vi "Readback Data_w_Waveform_no logging.vi"(0 "Semiconductor Module Context":T1, 5 "Pins":string[](array[string])=["CLK", "SDA"], 9 "Digital Format":string="RFFE6", 11 "error in (no error)":errorcluster, 12 "Register_Address_Dec":u8=80 format="%.0x", 13 "Bit_Location(LSB)":u8=7 max=7, 14 "#ofBits":u8=1 min=1 max=8) -> (4 "Reg Value":u8 format="%.0b", 15 "error out":errorcluster)   [LabVIEW 2013]
uses:
  <vilib>/NI_TestStand_SemiconductorModule/NI_TestStand_Semiconductor_Module.lvlibp/PinMap/General/SemiconductorModuleContext.ctl
  MIPI_RFFE/Ctrls/Configuration.ctl
  MIPI_RFFE/Ctrls/ClockDataChannels.ctl
  MIPI_RFFE/Ctrls/RegReadWrite.ctl
  <instrlib>/niHSDIO/niHSDIO.llb/niHSDIO_ctl Generation Mode Values (Ring).ctl
  <vilib>/NI_TestStand_SemiconductorModule/NI_TestStand_Semiconductor_Module.lvlibp/PinMap/HSDIO/PinsToNIHSDIOSessions.vi
  <vilib>/Waveform/DWDTOps.llb/DWDT Digital Size.vi
  <instrlib>/niHSDIO/niHSDIO.llb/niHSDIO Write Named Waveform (WDT).vi
  <instrlib>/niHSDIO/niHSDIO.llb/niHSDIO Fetch Waveform (WDT).vi
  <vilib>/NI_TestStand_SemiconductorModule/NI_TestStand_Semiconductor_Module.lvlibp
panel:
  out "Converted Data":T2 {"Register" max=31 format="%.0x"; "Slave Address" max=15 format="%.0x"}
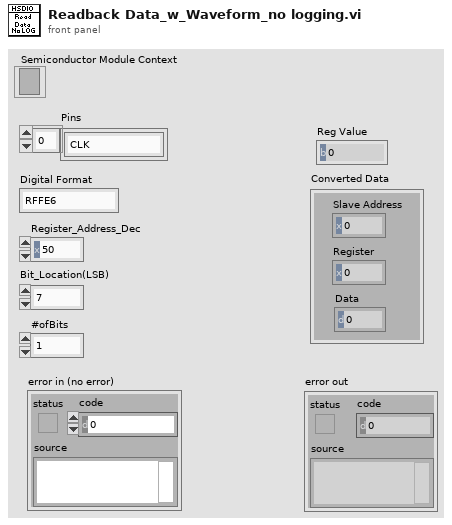
[diagram p1: front panel]
types:
  T1 = typedef "NI_TestStand_Semiconductor_Module.lvlibp/SemiconductorModuleContext.ctl" = refnum<k7>
  T2 = cluster{"Slave Address":u8, "Register":u8, "Data":u8}
  T3 = typedef "RegReadWrite.ctl" = cluster{"Slave Address":u8, "Register":u8, "Data":u8, "SetID_Pin_State":enum16{"0", "1", "Z"}}
  T4 = typedef "Configuration.ctl" = cluster{"Samples to Allocate":i32, "Oversample Factor":u8, "Clock Channel":T5, "Data Channel":T5}
  T5 = typedef "ClockDataChannels.ctl" = enum16{"0", "1"}
  T6 = typedef "niHSDIO_ctl Generation Mode Values (Ring).ctl" = i32
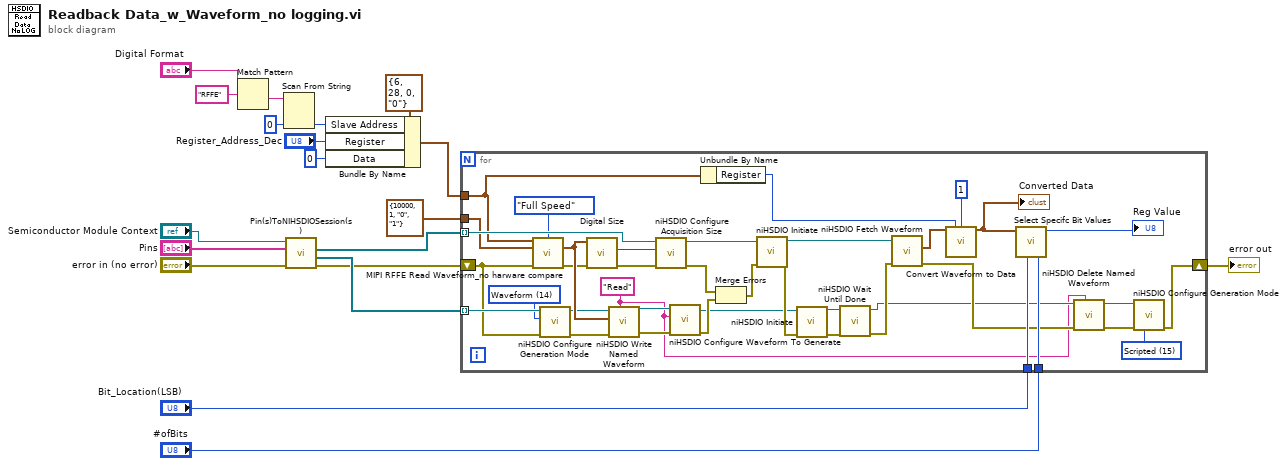
[diagram p0: block diagram]
diagram:
  n1 = Match Pattern(string="Digital Format", regular expression="RFFE") -> (after substring=w4:string)  [unwired: 1 in, 3 out]
  n2 = Scan From String(input string=w4, default 1=u8 0 ("Slave Address")) -> (output 1=w2:u8)  [unwired: 3 in, 3 out]
  n3 = call-poly <vilib>:"Pin(s)ToNIHSDIOSession(s).vi"("error in (no error)"="error in (no error)", "Pins"="Pins", "Semiconductor Module Context"="Semiconductor Module Context") -> ("error out"=w16:errorcluster, "Generation Sessions"=w17:refnum<k15>[], "Acquisition Sessions"=w18:refnum<k15>[])  [unwired: 3 in, 3 out]
  n4 = Bundle By Name(cluster=T3 {"Slave Address"=6, "Register"=28, "Data"=0, "SetID_Pin_State"=enum."0"} ("Data"), "Slave Address"=w2, "Register"="Register_Address_Dec", "Data"=u8 0) -> (w7:T3)
  n5 = for {
    tunnel: w18 -> [w48] mode=indexing
    tunnel: w17 -> [w38] mode=indexing
    tunnel: w7 -> [w27]
    tunnel: T4 {"Samples to Allocate"=10000, "Oversample Factor"=1, "Clock Channel"=enum."0", "Data Channel"=enum."1"} ("Configuratation") -> [w46]
    tunnel: "Bit_Location(LSB)" -> [w45]
    tunnel: "#ofBits" -> [w44]
    shift-right: [w29] -> w1
    shift-left: w16 -> [w35]
    w28 = T6 15 items=["Waveform"=14, "Scripted"=15] ("generation mode (waveform)")
    w20 = "Read" ("waveform name (default:\"\")")
    w34 = T6 14 items=["Waveform"=14, "Scripted"=15] ("generation mode (waveform)")
    n6 = call "MIPI RFFE Read Waveform_no harware compare.vi"("Data"=w27, "Readback Speed"=enum16{"Full Speed", "Half Speed"}."Full Speed", "Configuratation"=w46, "error in (no error)"=w35) -> ("Waveform Graph"=w53:digitalwaveform, "error out"=w50:errorcluster)  [unwired: 10 in]
    n7 = call <instrlib>:"niHSDIO Configure Generation Mode.vi"("error in (no error)"=w35, "generation mode (waveform)"=w34, "instrument handle"=w38) -> ("error out"=w36:errorcluster, "instrument handle out"=w37:refnum<k15>)  [unwired: 7 in]
    n8 = call-poly <vilib>:"Digital Size.vi"("error in (no error)"=w50, "digital waveform in"=w53) -> ("error out"=w51:errorcluster, "number of samples"=w52:i32)  [unwired: 6 in, 2 out]
    n9 = call-poly <instrlib>:"niHSDIO Write Named Waveform.vi"("waveform name (default:\"\")"=w20, "error in (no error)"=w36, "data"=w53, "instrument handle"=w37) -> ("error out"=w33:errorcluster, "instrument handle out"=w31:refnum<k15>)  [unwired: 6 in]
    n10 = call <instrlib>:"niHSDIO Configure Acquisition Size.vi"("error in (no error)"=w51, "samples per record (1000 samples)"=w52, "instrument handle"=w48) -> ("error out"=w47:errorcluster, "instrument handle out"=w55:refnum<k15>)  [unwired: 7 in]
    n11 = call <instrlib>:"niHSDIO Configure Waveform To Generate.vi"("error in (no error)"=w33, "waveform name"=w20, "instrument handle"=w31) -> ("error out"=w32:errorcluster, "instrument handle out"=w30:refnum<k15>)  [unwired: 7 in]
    n12 = Unbundle By Name(w27) -> ("Register"=w26:u8)
    n13 = Merge Errors(w47, w32) -> (w56:errorcluster)
    n14 = call <instrlib>:"niHSDIO Initiate.vi"("error in (no error)"=w56, "instrument handle"=w55) -> ("error out"=w58:errorcluster, "instrument handle out"=w39:refnum<k15>)  [unwired: 8 in]
    n15 = call <instrlib>:"niHSDIO Initiate.vi"("error in (no error)"=w58, "instrument handle"=w30) -> ("error out"=w57:errorcluster, "instrument handle out"=w40:refnum<k15>)  [unwired: 8 in]
    n16 = call <instrlib>:"niHSDIO Wait Until Done.vi"("error in (no error)"=w57, "instrument handle"=w40) -> ("error out"=w43:errorcluster, "instrument handle out"=w22:refnum<k15>)  [unwired: 8 in]
    n17 = call-poly <instrlib>:"niHSDIO Fetch Waveform.vi"("error in (no error)"=w43, "instrument handle"=w39) -> ("error out"=w24:errorcluster, "data"=w54:digitalwaveform)  [unwired: 6 in, 2 out]
    n18 = call "Convert Waveform to Data.vi"("Waveform Graph"=w54, "Register"=w26, "Ext_Read_Num_Reg"=u8 1) -> ("Converted Data"=w49:T2)  [unwired: 10 in, 2 out]
    "Converted Data" <- w49
    n19 = call "Select Specifc Bit Values.vi"("#ofBits"=w44, "Bit_Location(LSB)"=w45, "Converted Data"=w49) -> ("Bits"=→"Reg Value":u8)  [unwired: 8 in]
    n20 = call <instrlib>:"niHSDIO Delete Named Waveform.vi"("waveform name (default:\"\")"=w20, "error in (no error)"=w24, "instrument handle"=w22) -> ("error out"=w23:errorcluster, "instrument handle out"=w21:refnum<k15>)  [unwired: 7 in]
    n21 = call <instrlib>:"niHSDIO Configure Generation Mode.vi"("error in (no error)"=w23, "generation mode (waveform)"=w28, "instrument handle"=w21) -> ("error out"=w29:errorcluster)  [unwired: 7 in, 1 out]
  }
  "error out" <- w1
